vi "imaq get all keys and values.vi"(8 "error in (no error)":errorcluster, 11 "Refnum in":T1) -> (0 "error out":errorcluster, 1 "Key values":string[](array[string]), 2 "Keys":string[](array[string]), 3 "Refnum out":T1)   [LabVIEW 2020, in "Point Grey Camera.lvclass"]
uses:
  Point Grey Camera.lvclass
  IMAQ Image.ctl
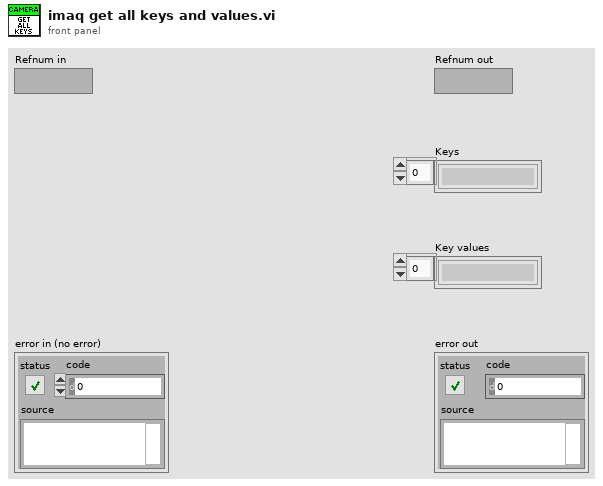
[diagram p1: front panel]
types:
  T1 = typedef "IMAQ Image.ctl" = refnum<image>
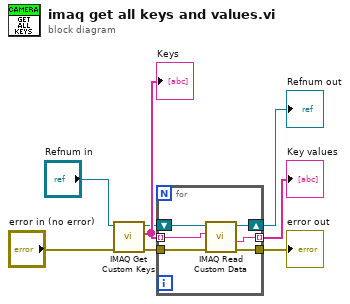
[diagram p0: block diagram]
diagram:
  n1 = call "IMAQ Get Custom Keys"("error in (no error)"="error in (no error)", "Image"="Refnum in") -> ("error out"=w7:errorcluster, "Keys"=w5:string[], "Image (duplicate)"=w3:T1)  [unwired: 6 in, 1 out]
  "Keys" <- w5
  n2 = for {
    shift-right: [w13] -> w4
    shift-left: w3 -> [w14]
    tunnel: w5 -> [w12] mode=indexing
    tunnel: [w11] -> w6 mode=indexing
    tunnel: w7 -> [w10]
    tunnel: [w9] -> w8
    n3 = call "IMAQ Read Custom Data"("error in (no error)"=w10, "Key"=w12, "Image"=w14) -> ("error out"=w9:errorcluster, "Custom Data Out"=w11:string, "Image (duplicate)"=w13:T1)  [unwired: 6 in]
  }
  "error out" <- w8
  "Key values" <- w6
  "Refnum out" <- w4
